vi "query.net.vi"(8 "错误输入（无错误）":errorcluster, 10 "Sql":string="SELECT * FROM vprojectTDR", 11 "DBSet":T1) -> (0 "错误输出":errorcluster, 3 "result":string[][](array[string]))   [LabVIEW 2011]
uses:
  System.Data
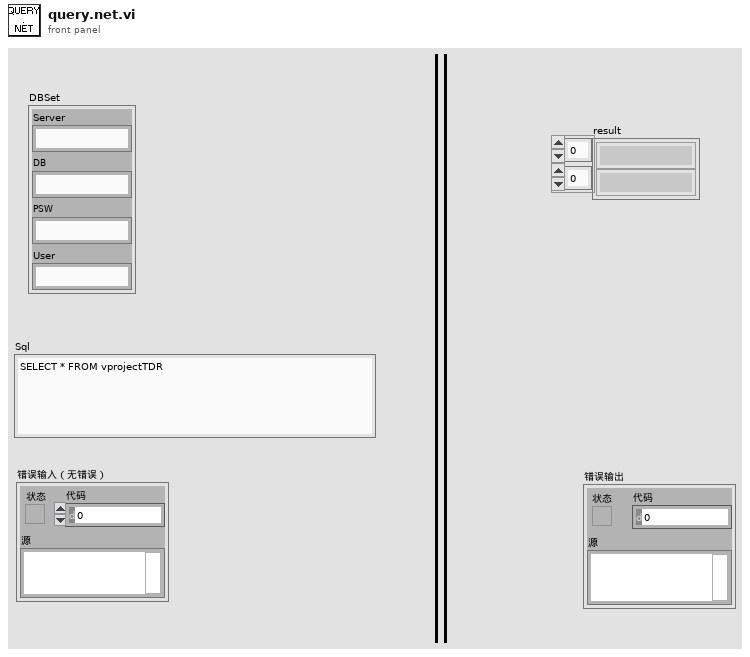
[diagram p1: front panel]
types:
  T1 = cluster{"Server":string, "DB":string, "PSW":string, "User":string}
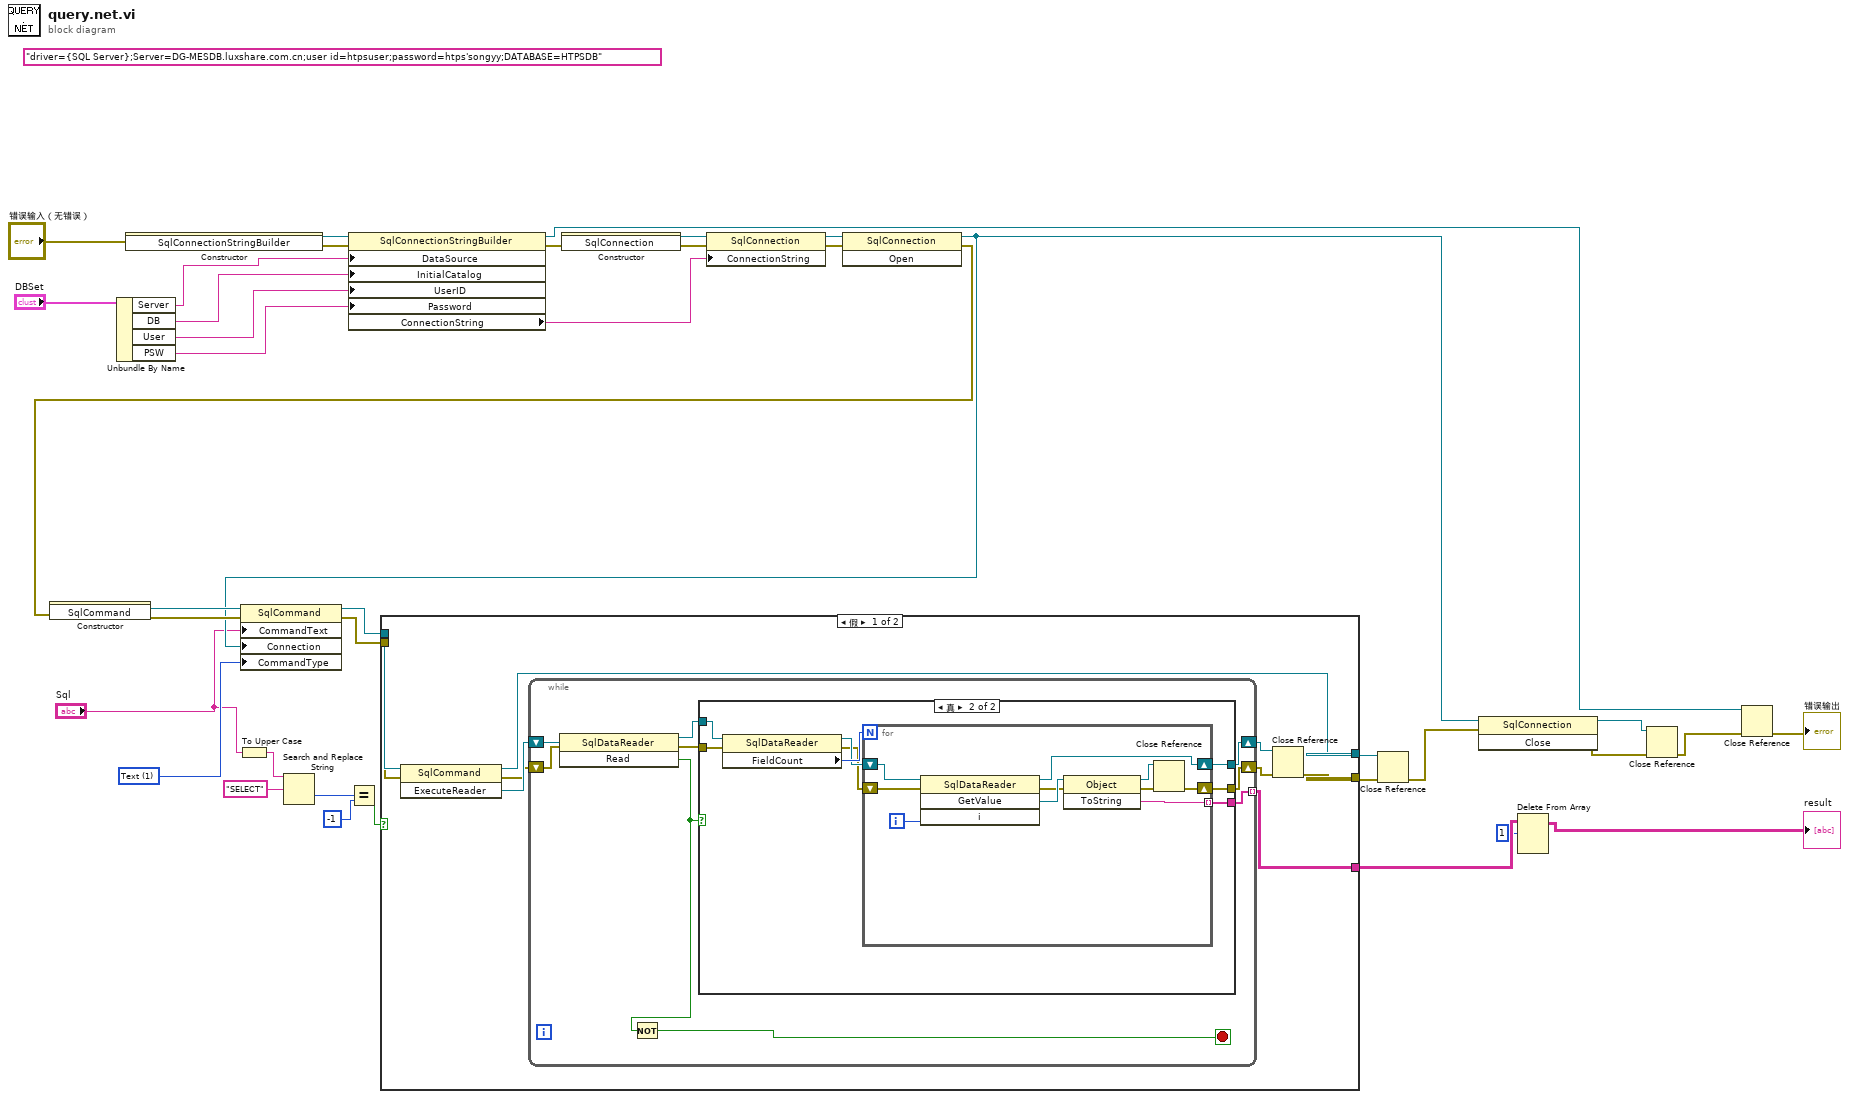
[diagram p0: block diagram]
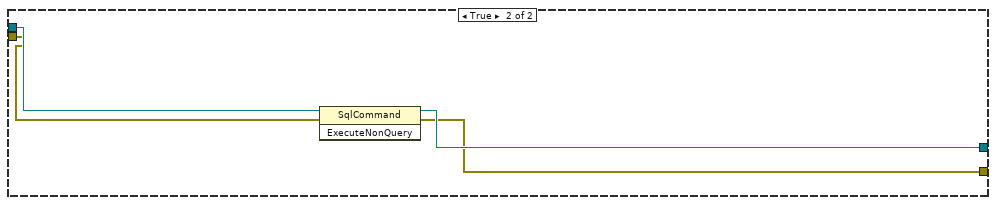
[diagram p3: hidden frame]
diagram:
  w33 = 1 items=["Text"=1, "StoredProcedure"=4, "TableDirect"=512] ("CommandType")
  (unwired) "driver={SQL Server};Server=DG-MESDB.luxshare.com.cn;user id=htpsuser;password=htps'songyy;DATABASE=HTPSDB" ("ConnectionString")
  n1 = Unbundle By Name("DBSet") -> ("Server"=w4:string, "DB"=w3:string, "User"=w2:string, "PSW"=w1:string)
  n2 = constructor class="SqlConnectionStringBuilder"(error in="错误输入（无错误）") -> (reference out=w36:refnum<k24>, error out=w30:errorcluster)  [unwired: 2 in, 1 out]
  n3 = To Upper Case(1:"Sql") -> (0:w14:string)
  n4 = Search and Replace String(input string=w14, search string="SELECT" ("搜索字符串")) -> (offset past replacement=w12:i32)  [unwired: 6 in, 3 out]
  n5 = property class="SqlConnectionStringBuilder"(reference=w36, error in=w30, "DataSource"=w4, "InitialCatalog"=w3, "UserID"=w2, "Password"=w1) -> (reference out=w19:refnum<k24>, error out=w29:errorcluster, "ConnectionString"=w35:string)
  n6 = Equal?(x=w12, y=-1) -> (x = y?=w10:bool)
  n7 = constructor class="SqlConnection"(error in=w29) -> (reference out=w38:refnum<k24>, error out=w28:errorcluster)  [unwired: 2 in, 1 out]
  n8 = property class="SqlConnection"(reference=w38, error in=w28, "ConnectionString"=w35) -> (reference out=w37:refnum<k24>, error out=w27:errorcluster)
  n9 = invoke class="SqlConnection" method="Open"(reference=w37, error in=w27) -> (reference out=w23:refnum<k24>, error out=w26:errorcluster)  [unwired: 1 in, 1 out]
  n10 = constructor class="SqlCommand"(error in=w26) -> (reference out=w34:refnum<k24>, error out=w25:errorcluster)  [unwired: 2 in, 1 out]
  n11 = property class="SqlCommand"(reference=w34, error in=w25, "CommandText"="Sql", "Connection"=w23, "CommandType"=w33) -> (reference out=w32:refnum<k24>, error out=w24:errorcluster)
  n12 = case shown="假" w10 {
    tunnel: w32 -> [w47 w80]
    tunnel: [w46 _] -> w8
    tunnel: w24 -> [w45 w79]
    tunnel: [w40 w78] -> w17
    tunnel: [w39 w77] -> w16
    frame False {
      n13 = invoke class="SqlCommand" method="ExecuteReader"(reference=w47, error in=w45) -> (reference out=w40:refnum<k24>, error out=w43:errorcluster, "ExecuteReader"=w44:refnum<k24>)  [unwired: 1 in]
      n14 = while {
        shift-right: [w53] -> w42
        shift-left: w44 -> [w56]
        tunnel: [w54] -> w46 mode=indexing
        shift-right: [w50] -> w41
        shift-left: w43 -> [w52]
        stop <- w48 stop-if-true
        n15 = invoke class="SqlDataReader" method="Read"(reference=w56, error in=w52) -> (reference out=w55:refnum<k24>, error out=w51:errorcluster, "Read"=w49:bool)  [unwired: 1 in]
        n16 = Not(x=w49) -> (.not. x?=w48:bool)
        n17 = case shown="真" w49 {
          tunnel: w55 -> [w58 w66]
          tunnel: [_ w63] -> w54
          tunnel: [w58 w62] -> w53
          tunnel: w51 -> [w57 w61]
          tunnel: [w57 w59] -> w50
          frame False {
          }
          frame True {
            n18 = property class="SqlDataReader"(reference=w66, error in=w61) -> (reference out=w64:refnum<k24>, error out=w60:errorcluster, "FieldCount"=w65:i32)
            n19 = for {
              N: w65 -> [_]
              tunnel: [w74] -> w63 mode=indexing
              shift-right: [w72] -> w62
              shift-left: w64 -> [w73]
              shift-right: [w67] -> w59
              shift-left: w60 -> [w71]
              i -> [w76]
              n20 = invoke class="SqlDataReader" method="GetValue"(reference=w73, error in=w71, "i"=w76) -> (reference out=w72:refnum<k24>, error out=w70:errorcluster, "GetValue"=w75:refnum<k24>)  [unwired: 1 in, 1 out]
              n21 = invoke class="Object" method="ToString"(reference=w75, error in=w70) -> (reference out=w69:refnum<k24>, error out=w68:errorcluster, "ToString"=w74:string)  [unwired: 1 in]
              n22 = Close Reference(reference=w69, error in (no error)=w68) -> (error out=w67:errorcluster)
            }
          }
        }
      }
      n23 = Close Reference(reference=w42, error in (no error)=w41) -> (error out=w39:errorcluster)
    }
    frame True {
      n24 = invoke class="SqlCommand" method="ExecuteNonQuery"(reference=w80, error in=w79) -> (reference out=w78:refnum<k24>, error out=w77:errorcluster)  [unwired: 1 in, 1 out]
    }
  }
  n25 = Close Reference(reference=w17, error in (no error)=w16) -> (error out=w22:errorcluster)
  n26 = invoke class="SqlConnection" method="Close"(reference=w23, error in=w22) -> (reference out=w21:refnum<k24>, error out=w20:errorcluster)  [unwired: 1 in, 1 out]
  n27 = Delete From Array(array=w8, length=1 ("长度")) -> (array with subset deleted=→"result":string[][])  [unwired: 2 in, 1 out]
  n28 = Close Reference(reference=w21, error in (no error)=w20) -> (error out=w18:errorcluster)
  n29 = Close Reference(reference=w19, error in (no error)=w18) -> (error out=→"错误输出":errorcluster)
